vi "model-wrapper -- analytic derivatives -- grad and curvature -- V6.vi"(5 "model":T1, 7 "action":T3=enum."onlygrads", 8 "parameters map  IN":map{T2, dbl}(c390), 10 "ω (rad/sec)":dbl=0.1 format="%#_10f") -> (0 "parameters map  OUT":map{T2, dbl}(c390), 1 "λdζ(ω)/dλ OUT":map{T2, cdb}(c390), 2 "ω out (rad/sec)":dbl=0.1 format="%#_10f", 3 "ζ(ω) OUT":cdb=0.1+0.0i format="%#_10f")   [LabVIEW 2021]
uses:
  3-lorentzian-heat-response action.ctl
  3-lorentzian-parameters.ctl
  spectral model.ctl
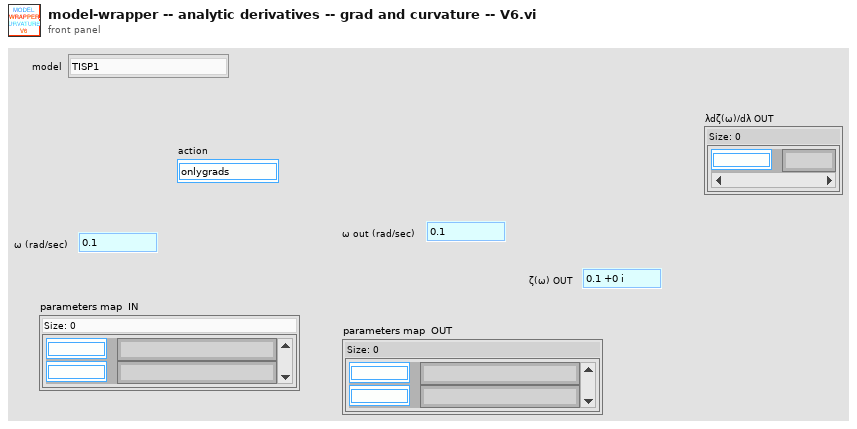
[diagram p1: front panel]
types:
  T1 = typedef "spectral model.ctl" = enum16{"TISP1", "stanford1"}
  T2 = typedef "3-lorentzian-parameters.ctl" = enum16{"ζ", "τ1", "τS", "τN", "τC", "κ0", "m1", "m2", "m3", "T (K)", "B (T)", "θ (deg)", "side (S|R)", "set of (B|T)", "Re(offset)", "Im(offset)", "στ1", "στ1-", "στ1+", "στS", "στS-", "στS+", "στN", "στN-", "στN+", "τ11", "τ12", "τ21", "τ22", "τN1", "τN2", "σηlogτ1", "σηlogτS", "σηlogτN", "σlogτ1", "σlogτS", "σlogτN", "σητ1", "σητS", "σητN", "noiseT", "plain", "vproj"}
  T3 = typedef "3-lorentzian-heat-response action.ctl" = enum16{"calc R", "create string", "calc m1m2m3", "dζ", "dT1", "dτS", "dτN", "dτC", "d-all", "dκ0", "T(K)", "m1", "m2", "m3", "parse string", "θ (deg)", "B (T)", "onlygrads", "newton", "create emty string", "simple2nd", "calc R2", "ScalarProd", "ScalarProd-diff", "nothing", "ScalarProd-eta", "tolog", "ignore", "three2nd", "eta-errors"}
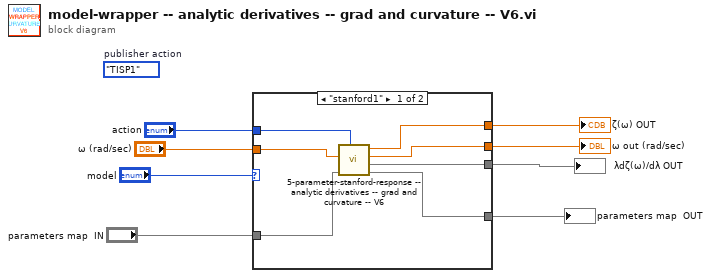
[diagram p0: block diagram]
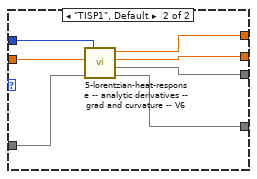
[diagram p2: hidden frame]
diagram:
  (unwired) spectral_model."TISP1"  # publisher action
  n1 = case shown="\"stanford1\"" "model" {
    tunnel: "ω (rad/sec)" -> [w14 w21]
    tunnel: [w15 w16] -> w6
    tunnel: "parameters map  IN" -> [w13 w20]
    tunnel: "action" -> [w12 w22]
    tunnel: [w11 w19] -> w3
    tunnel: [w10 w17] -> w2
    tunnel: [w9 w18] -> w1
    frame "stanford1" {
      n2 = call "5-parameter-stanford-response -- analytic derivatives -- grad and curvature -- V6.vi"("action"=w12, "parameters map  IN"=w13, "ω (rad/sec)"=w14) -> ("parameters map  OUT"=w11:map{T2, dbl}, "λdζ(ω)/dλ OUT"=w9:map{T2, cdb}, "ω out (rad/sec)"=w15:dbl, "ζ(ω) OUT"=w10:cdb)  [unwired: 5 in]
    }
    frame "TISP1", Default {
      n3 = call "5-lorentzian-heat-response -- analytic derivatives -- grad and curvature -- V6.vi"("action"=w22, "parameters map  IN"=w20, "ω (rad/sec)"=w21) -> ("parameters map  OUT"=w19:map{T2, dbl}, "λdζ(ω)/dλ OUT"=w18:map{T2, cdb}, "ω out (rad/sec)"=w16:dbl, "ζ(ω) OUT"=w17:cdb)  [unwired: 5 in]
    }
  }
  "ζ(ω) OUT" <- w2
  "ω out (rad/sec)" <- w6
  "parameters map  OUT" <- w3
  "λdζ(ω)/dλ OUT" <- w1
